vi "Actor Core.vi"(8 "error in":errorcluster, 11 "Worker in":refnum<class "Worker.lvclass">) -> (0 "error out":errorcluster, 3 "Actor out":refnum<class "Actor.lvclass">)   [LabVIEW 2023, in "Worker.lvlib" / "Worker.lvclass"]
doc: "(<B>Filename</B>: Actor Framework.lvlib:Actor.lvclass:Actor Core.vi)\n\nReceives messages to the actor, reacts to them, and initiates any error handling that may shut the actor down.\n\nDescendant classes may override this VI to append parallel tasks for the actor to complete while it handles messages. Overrides use the Call Parent Method node."
uses:
  Worker.lvclass
  c:/dev/_r/4/eng/lv-core/lvpostprocessingd/lv_mc_x86_64/dist_i386/vi.lib/ActorFramework/Actor/Actor.lvclass
  <vilib>/ActorFramework/Actor/Actor.lvclass
  <vilib>/ActorFramework/Actor/Actor.lvclass/Actor.ctl
  <vilib>/ActorFramework/Message Enqueuer/Message Enqueuer.lvclass/Message Enqueuer.ctl
  Worker.lvclass/Worker.ctl
  Person Messages/Show or Hide Front Panel Msg/Show or Hide Front Panel Msg.lvclass/Show or Hide Front Panel Msg.ctl
  Coffee Shop/Entity Types.ctl
  Coffee Shop Messages/Update Entity Details Msg/Update Entity Details Msg.lvclass/Update Entity Details Msg.ctl
  Work Dispatcher Messages/Add Available Worker Msg/Add Available Worker Msg.lvclass/Add Available Worker Msg.ctl
  <vilib>/ActorFramework/Message Enqueuer/Init from Existing Queue.vi
  <vilib>/ActorFramework/Message Enqueuer/Enqueue.vi
  Person Messages/Show or Hide Front Panel Msg/Show or Hide Front Panel Msg.lvclass
  c:/dev/_r/4/eng/lv-core/lvpostprocessingd/lv_mc_x86_64/dist_i386/vi.lib/ActorFramework/Message/Message.lvclass
  Coffee Shop Messages/Update Entity Details Msg/Update Entity Details Msg.lvclass
  Work Dispatcher Messages/Add Available Worker Msg/Add Available Worker Msg.lvclass
  <vilib>/ActorFramework/Message Priority Queue/Priority Enqueue.vi
  <vilib>/ActorFramework/Message Enqueuer/Message Enqueuer.lvclass
  Person/Person.lvclass
  Coffee Shop/Coffee Shop.lvclass
panel:
  out "Name":string
  out "Worker Type":string="Barista"
  out "Orders Filled This Shift":dbl
  out "Status":string="Waiting..."
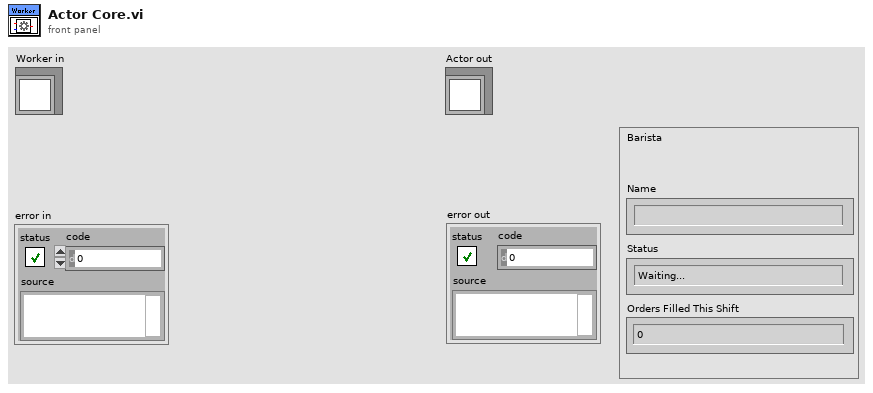
[diagram p1: front panel]
types:
  T1 = typedef "Coffee Shop.lvlib/Coffee Shop.lvclass/Entity Types.ctl" = enum16{"Customer", "Cashier", "Barista"}
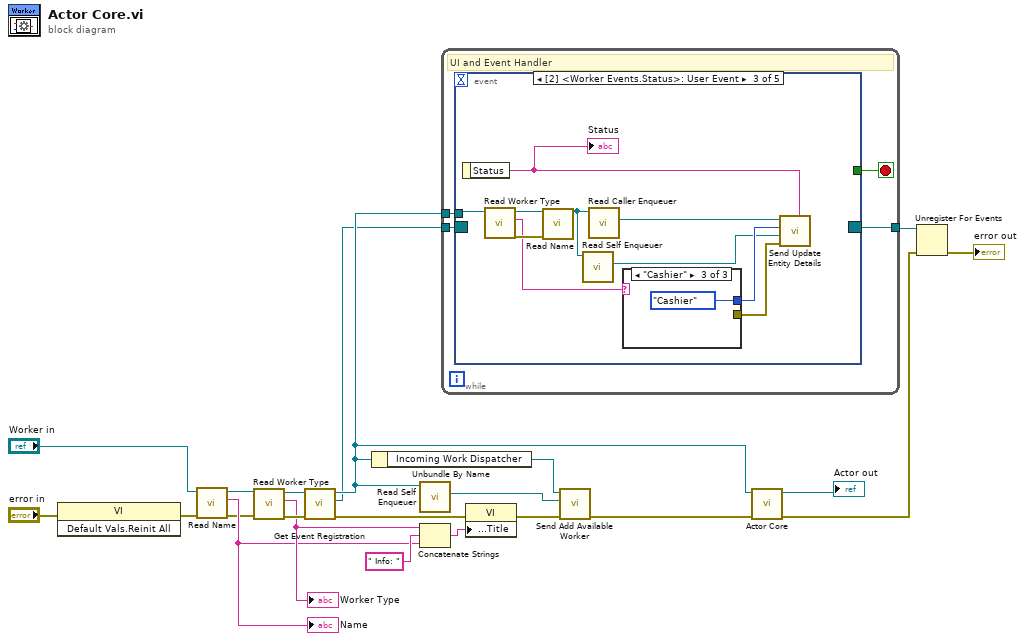
[diagram p0: block diagram]
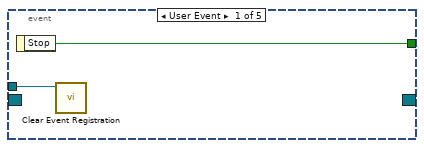
[diagram p2: hidden frame]
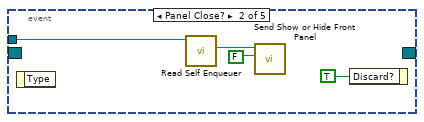
[diagram p3: hidden frame]
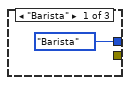
[diagram p4: hidden frame]
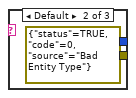
[diagram p5: hidden frame]
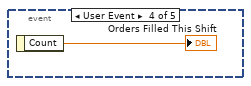
[diagram p6: hidden frame]
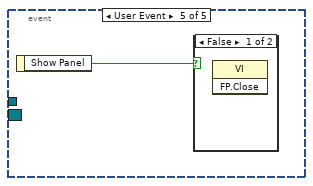
[diagram p7: hidden frame]
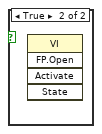
[diagram p8: hidden frame]
diagram:
  n1 = invoke on="Invoke Node" class="VI" method="Default Vals.Reinit All"(error in="error in") -> (error out=w1:errorcluster)  [unwired: 2 in, 2 out]
  n2 = call-dynamic "Read Name.vi"("error in (no error)"=w1, "Person in"="Worker in") -> ("error out"=w3:errorcluster, "Name"=w8:string, "Person out"=w2:refnum<class "Worker.lvclass">)  [unwired: 7 in]
  "Name" <- w8
  n3 = call-dynamic "Read Worker Type.vi"("error in (no error)"=w3, "Worker in"=w2) -> ("error out"=w16:errorcluster, "Type"=w10:string, "Worker out"=w17:refnum<class "Worker.lvclass">)  [unwired: 7 in]
  "Worker Type" <- w10
  n4 = call-dynamic "Get Event Registration.vi"("error in (no error)"=w16, "Worker in"=w17) -> ("error out"=w11:errorcluster, "Event Registration Refnum"=w18:refnum<event-registration>, "Worker out"=w19:refnum<class "Worker.lvclass">)  [unwired: 7 in]
  n5 = Unbundle By Name(w19) -> ("Incoming Work Dispatcher"=w22:refnum<class "Message Enqueuer.lvclass">)
  n6 = call <vilib>:"Read Self Enqueuer.vi"("Actor"=w19) -> ("Self Enqueuer"=w21:refnum<class "Message Enqueuer.lvclass">)  [unwired: 10 in]
  n7 = Concatenate Strings(w10, " Info: " ("format string"), w8) -> (w12:string)
  n8 = while {
    tunnel: w18 -> [w26]
    tunnel: w19 -> [w24]
    tunnel: [w23] -> w7
    stop <- w25 stop-if-true
    # "UI and Event Handler"
    n9 = event shown="[2] <Worker Events.Status>: User Event" {
      selector: w26 -> [_ _ _ _ _]
      dyn-events: [_ _ _ _ _] -> w23
      timeout: _ -> [_ _ _ _ _]
      tunnel: [w28 _ _ _ _] -> w25
      tunnel: w24 -> [w27 w32 w40 _ _]
      event User Event {
        n10 = event-data() -> ("Stop"=w28:bool)  [unwired: 1 in]
        n11 = call-dynamic "Clear Event Registration.vi"("Worker in"=w27) -> ()  [unwired: 9 in, 2 out]
      }
      event Panel Close? {
        n12 = event-data() -> ()  [unwired: 1 in, 1 out]
        n13 = call <vilib>:"Read Self Enqueuer.vi"("Actor"=w32) -> ("Self Enqueuer"=w31:refnum<class "Message Enqueuer.lvclass">)  [unwired: 10 in]
        n14 = call "Send Show or Hide Front Panel.vi"("Show Front Panel?"=FALSE, "Message Enqueuer"=w31) -> ()  [unwired: 8 in, 2 out]
        n15 = event-data ("Event Filter Node")("Discard?"=TRUE) -> ()  [unwired: 1 in, 1 out]
      }
      event User Event {
        n16 = event-data() -> ("Status"=w33:string)  [unwired: 1 in]
        "Status" <- w33
        n17 = call-dynamic "Read Worker Type.vi"("Worker in"=w40) -> ("error out"=w38:errorcluster, "Type"=w36:string, "Worker out"=w39:refnum<class "Worker.lvclass">)  [unwired: 8 in]
        n18 = call-dynamic "Read Name.vi"("error in (no error)"=w38, "Person in"=w39) -> ("Person out"=w41:refnum<class "Worker.lvclass">)  [unwired: 7 in, 2 out]
        n19 = call <vilib>:"Read Self Enqueuer.vi"("Actor"=w41) -> ("Self Enqueuer"=w34:refnum<class "Message Enqueuer.lvclass">)  [unwired: 10 in]
        n20 = call <vilib>:"Read Caller Enqueuer.vi"("Actor"=w41) -> ("Caller Enqueuer"=w42:refnum<class "Message Enqueuer.lvclass">)  [unwired: 10 in]
        n21 = case shown="\"Cashier\"" w36 {
          tunnel: [Entity_Types."Barista" ("Entity Type") _ Entity_Types."Cashier" ("Entity Type")] -> w37
          tunnel: [_ errorcluster {"status"=TRUE, "code"=0, "source"="Bad Entity Type"} ("error constant") _] -> w35
          frame "Barista" {
          }
          frame Default {
          }
          frame "Cashier" {
          }
        }
        n22 = call "Send Update Entity Details.vi"("status"=w33, "error in (no error)"=w35, "enqueuer"=w34, "Entity Type"=w37, "Message Enqueuer"=w42) -> ()  [unwired: 5 in, 2 out]
      }
      event User Event {
        n23 = event-data() -> ("Count"=→"Orders Filled This Shift":dbl)  [unwired: 1 in]
      }
      event User Event {
        n24 = event-data() -> ("Show Panel"=w47:bool)  [unwired: 1 in]
        n25 = case shown="False" w47 {
          frame False {
            n26 = invoke on="Invoke Node" class="VI" method="FP.Close"() -> ()  [unwired: 3 in, 3 out]
          }
          frame True {
            n27 = invoke on="Invoke Node" class="VI" method="FP.Open"() -> ()  [unwired: 5 in, 5 out]
          }
        }
      }
    }
  }
  n28 = property on="Property Node" class="VI"(error in=w11, "Front Panel.Title"=w12) -> (error out=w13:errorcluster)  [unwired: 1 in, 1 out]
  n29 = call "Send Add Available Worker.vi"("error in (no error)"=w13, "Worker"=w21, "Message Enqueuer"=w22) -> ("error out"=w20:errorcluster)  [unwired: 7 in, 1 out]
  n30 = call-parent "Actor Core.vi"("error in"=w20, "Actor in"=w19) -> ("error out"=w6:errorcluster, "Actor out"=→"Actor out":refnum<class "Actor.lvclass">)  [unwired: 8 in]
  n31 = Unregister For Events(event registration refnum=w7, error in=w6) -> (error out=→"error out":errorcluster)
